vi "Calculate Temperature.vi"(11 "Bytes Read":u8[](array[numeric])) -> (3 "Temp Deg C":dbl)   [LabVIEW 2017]
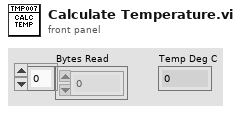
[diagram p1: front panel]
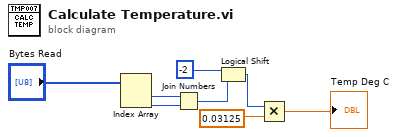
[diagram p0: block diagram]
diagram:
  n1 = Index Array(array="Bytes Read") -> (element #1=w3:u8, element #2=w4:u8)  [unwired: 2 in]
  n2 = Join Numbers(hi=w3, lo=w4) -> ((hi.lo)=w6:u16)
  n3 = Logical Shift(y=-2, x=w6) -> (x << y=w7:u16)
  n4 = Multiply(x=w7, y=0.03125) -> (x*y=→"Temp Deg C":dbl)
